vi "Global Setup.vi"(8 "error in (no error)":errorcluster, 11 "Global Fixture Template In":refnum<class "Global Fixture Template.lvclass">) -> (0 "error out":errorcluster)   [LabVIEW 2020, in "Global Fixture Template.lvclass"]
uses:
  Global Fixture Template.lvclass
  Global Fixture Template.lvclass/Global Fixture Template.ctl
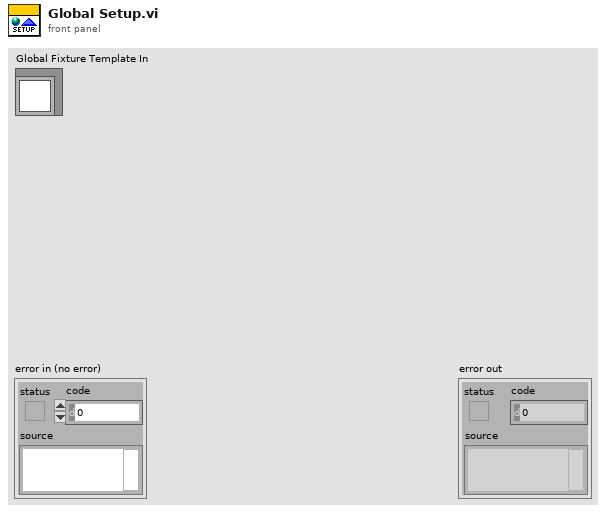
[diagram p1: front panel]
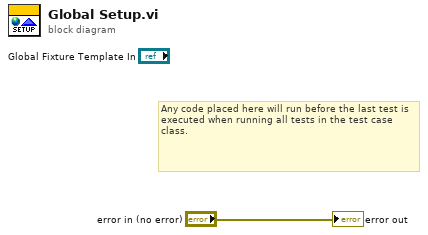
[diagram p0: block diagram]
diagram:
  # "Any code placed here will run before the last test is executed when running all tests in the test case class."
  "error out" <- "error in (no error)"
